vi "CMD_INVERT.vi"(8 "error in (no error)":errorcluster, 10 "Arguments":string[](array[string]), 11 "gScript Interpreter in":refnum<class "gScript Interpreter.lvclass">) -> (0 "error out":errorcluster, 3 "gScript Interpreter out":refnum<class "gScript Interpreter.lvclass">)   [LabVIEW 2017, in "gScript Interpreter.lvclass"]
uses:
  gScript Interpreter.lvclass
  Shared Components/Orient3d Class/Orient3d.lvclass
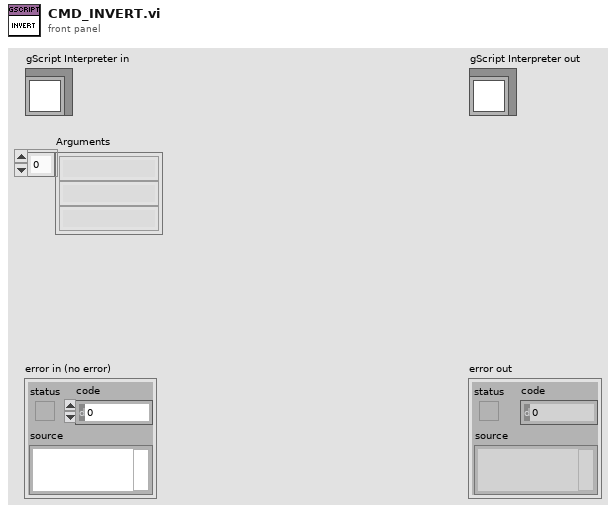
[diagram p1: front panel]
types:
  T1 = typedef "Memory Cell.ctl" = cluster{"type":T2, "x":dbl, "y":dbl, "z":dbl, "w":dbl}
  T2 = typedef "Memory Cell Type Enum.ctl" = enum16{"integer", "float", "vector", "rotation"}
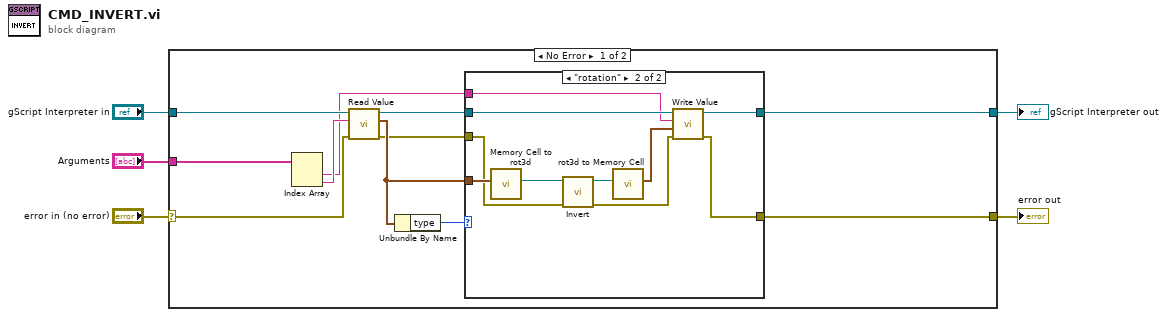
[diagram p0: block diagram]
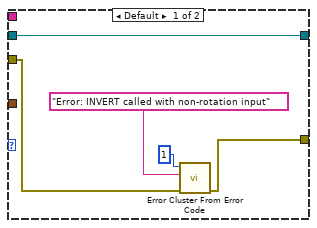
[diagram p2: hidden frame]
diagram:
  n1 = case shown="No Error" "error in (no error)" {
    selector: "error in (no error)" -> [w14 w33]
    tunnel: [w10 w33] -> w4
    tunnel: [w11 w32] -> w2
    tunnel: "gScript Interpreter in" -> [w15 w32]
    tunnel: "Arguments" -> [w16 _]
    frame No Error {
      n2 = Index Array(array=w16) -> (element #1=w12:string, element #2=w13:string)  [unwired: 2 in]
      n3 = call-dynamic "Read Value.vi"("error in (no error)"=w14, "String in"=w13, "gScript Interpreter in"=w15) -> ("error out"=w7:errorcluster, "Memory Cell"=w9:T1, "gScript Interpreter out"=w8:refnum<class "gScript Interpreter.lvclass">)  [unwired: 6 in]
      n4 = Unbundle By Name(w9) -> ("type"=w6:T2)
      n5 = case shown="\"rotation\"" w6 {
        tunnel: w8 -> [w21 w31]
        tunnel: w12 -> [_ w30]
        tunnel: w7 -> [w18 w24]
        tunnel: [w21 w29] -> w11
        tunnel: [w17 w28] -> w10
        tunnel: w9 -> [_ w27]
        frame Default {
          n6 = call <vilib>:"Error Cluster From Error Code.vi"("error in (no error)"=w18, "error message (\"\")"="Error: INVERT called with non-rotation input" ("error message (\"\")"), "error code (0)"=1) -> ("error out"=w17:errorcluster)  [unwired: 6 in]
        }
        frame "rotation" {
          n7 = call "Memory Cell to rot3d.vi"("Memory Cell"=w27) -> ("Orient3d out"=w25:refnum<class "Orient3d.lvclass">)  [unwired: 10 in]
          n8 = call "Invert.vi"("error in"=w24, "Orient3d in"=w25) -> ("error out"=w23:errorcluster, "Orient3d out"=w22:refnum<class "Orient3d.lvclass">)  [unwired: 8 in]
          n9 = call "rot3d to Memory Cell.vi"("Orient3d in"=w22) -> ("Memory Cell"=w26:T1)  [unwired: 10 in]
          n10 = call-dynamic "Write Value.vi"("error in (no error)"=w23, "Value"=w26, "Address"=w30, "gScript Interpreter in"=w31) -> ("error out"=w28:errorcluster, "gScript Interpreter out"=w29:refnum<class "gScript Interpreter.lvclass">)  [unwired: 6 in]
        }
      }
    }
    frame Error {
    }
  }
  "error out" <- w4
  "gScript Interpreter out" <- w2
